vi "Example.vi"() -> ()   [LabVIEW 2021, in "Tree.lvlib"]
uses:
  Tree.lvlib
  Tree.lvclass
panel:
  in  "Show Hierarhy":T1={"Show hierarhy in first column(F)"=TRUE, "Left separator"="", "Right separator"="/"}
  in  "Column":i32=2
  in  "Clear":bool
  in  "InsertPath":bool
  in  "InsertClass":bool
  in  "InsertPane":bool
  out "Random to variant":dbl
  in  "Strings":string[](array[string])
  in  "Edit":bool
  out "Selected Element":T2
  in  "Variant":variant
  in  "InsertClaster":bool
  in  "Filter":string
  in  "StepForward":bool
  in  "StepBack":bool
  in  "Child?":bool
  in  "Delete":bool
  in  "New Tag":string
  in  "Strings":string[](array[string])
  in  "Add":bool
  in  "stop":bool
  in  "Tree":string[](tree)
  # "Tree v0.2"
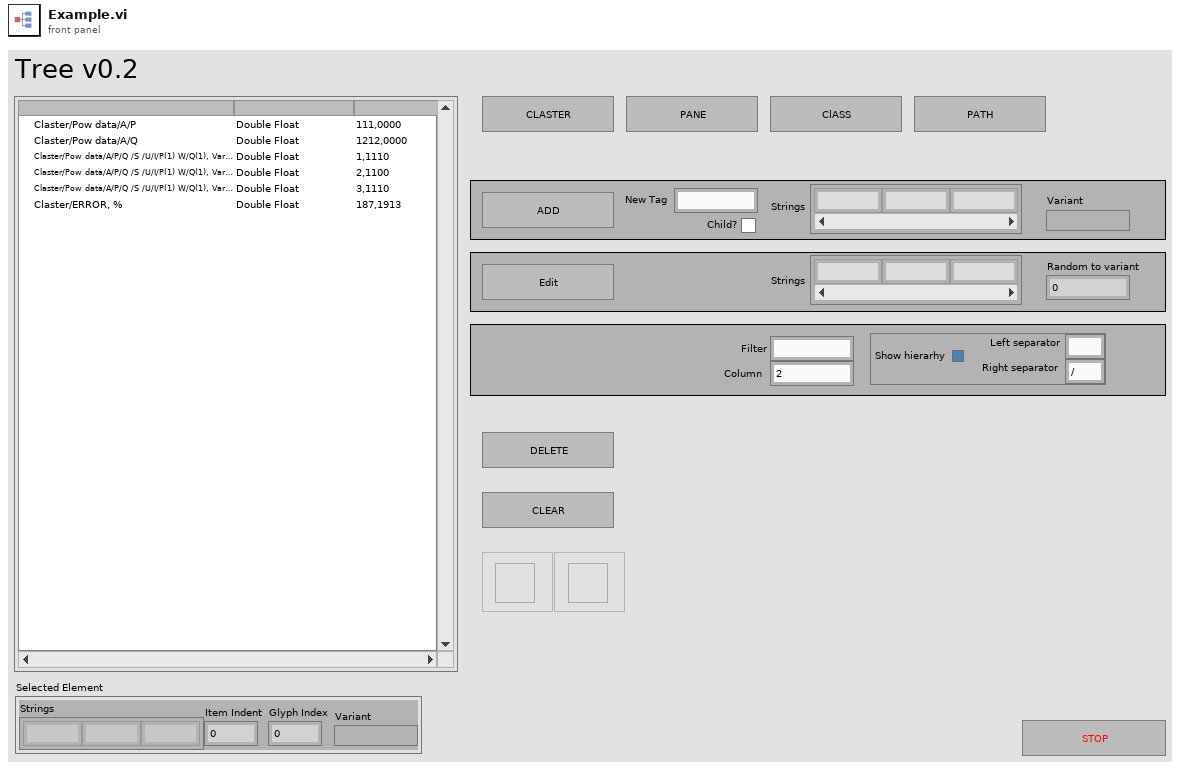
[diagram p1: front panel]
types:
  T1 = cluster{"Show hierarhy in first column(F)":bool, "Left separator":string, "Right separator":string}
  T2 = cluster{"Strings":string[], "Item Indent":i32, "Glyph Index":i32, "Variant":variant}
  T3 = enum16{"Clear & Insert", "Update Existing", "Add to End"}
  T4 = enum8{"Enabled", "Disabled", "Disabled and Grayed Out"}
  T5 = cluster{"Tag":string, "Strings":string[], "Open?":bool, "Item Indent":i32, "Glyph Index":i32, "Variant":variant}[]
  T6 = cluster{string, "New Tag":string, "Strings":string[], "Child?":bool, "Variant":variant}
  T7 = cluster{"Strings":string[], "Indent":i32, "Glyph Index":i32, "Variant":variant}
  T8 = cluster{"Pow data":cluster{"A":cluster{"P":dbl, "Q ":dbl, "S ":dbl, "U":dbl, "I":dbl, "P(1) W":dbl, "Q(1), Var":dbl, "S(1), VA":dbl, "cos(fi)":dbl, "sin(fi)":dbl, "Pow coef":string}, "B":cluster{"P":dbl, "Q ":dbl, "S ":dbl, "U":dbl, "I":dbl, "P(1) W":dbl, "Q(1), Var":dbl, "S(1), VA":dbl, "cos(fi)":dbl, "sin(fi)":dbl, "Pow coef":string}, "C":cluster{"P":dbl, "Q ":dbl, "S ":dbl, "U":dbl, "I":dbl, "P(1) W":dbl, "Q(1), Var":dbl, "S(1), VA":dbl, "cos(fi)":dbl, "sin(fi)":dbl, "Pow coef":string}, "N":cluster{"P":dbl, "Q ":dbl, "S ":dbl, "U":dbl, "I":dbl, "P(1) W":dbl, "Q(1), Var":dbl, "S(1), VA":dbl, "cos(fi)":dbl, "sin(fi)":dbl, "Pow coef":string}}, "Main data":cluster{"U":cluster{"RMS":cluster{"A":dbl, "B":dbl, "C":dbl, "N":dbl}, "DC":cluster{"A":dbl, "B":dbl, "C":dbl, "N":dbl}, "F(1)":cluster{"A":dbl, "B":dbl, "C":dbl, "N":dbl}, "RMS(1)":cluster{"A":dbl, "B":dbl, "C":dbl, "N":dbl}, "Phi":cluster{"A":dbl, "B":dbl, "C":dbl, "N":dbl}, "THD":cluster{"A":dbl, "B":dbl, "C":dbl, "N":dbl}}, "I":cluster{"RMS":cluster{"A":dbl, "B":dbl, "C":dbl, "N":dbl}, "DC":cluster{"A":dbl, "B":dbl, "C":dbl, "N":dbl}, "F(1)":cluster{"A":dbl, "B":dbl, "C":dbl, "N":dbl}, "RMS(1)":cluster{"A":dbl, "B":dbl, "C":dbl, "N":dbl}, "Phi":cluster{"A":dbl, "B":dbl, "C":dbl, "N":dbl}, "THD":cluster{"A":dbl, "B":dbl, "C":dbl, "N":dbl}}}, "Line voltage":cluster{"AB":dbl, "BC":dbl, "CA":dbl}, "Cref":dbl, "Nref_calc":dbl, "Ref Range":cluster{"I range":u8, "U range":u8}, "F out":cluster{"integer part":u32, "fractional part":u8}, "Ndut_culc_type":enum16{"Auto", "Ndut", "Tdut"}, "Ndut_calc":u32, "Tdut_calc":dbl, "ERROR, %":dbl, "Koef":u16, "Params 0xC5":cluster{"DUT_N":u32, "REF_N":u32, "REF_N 2":u32, "Iterations":u32}}
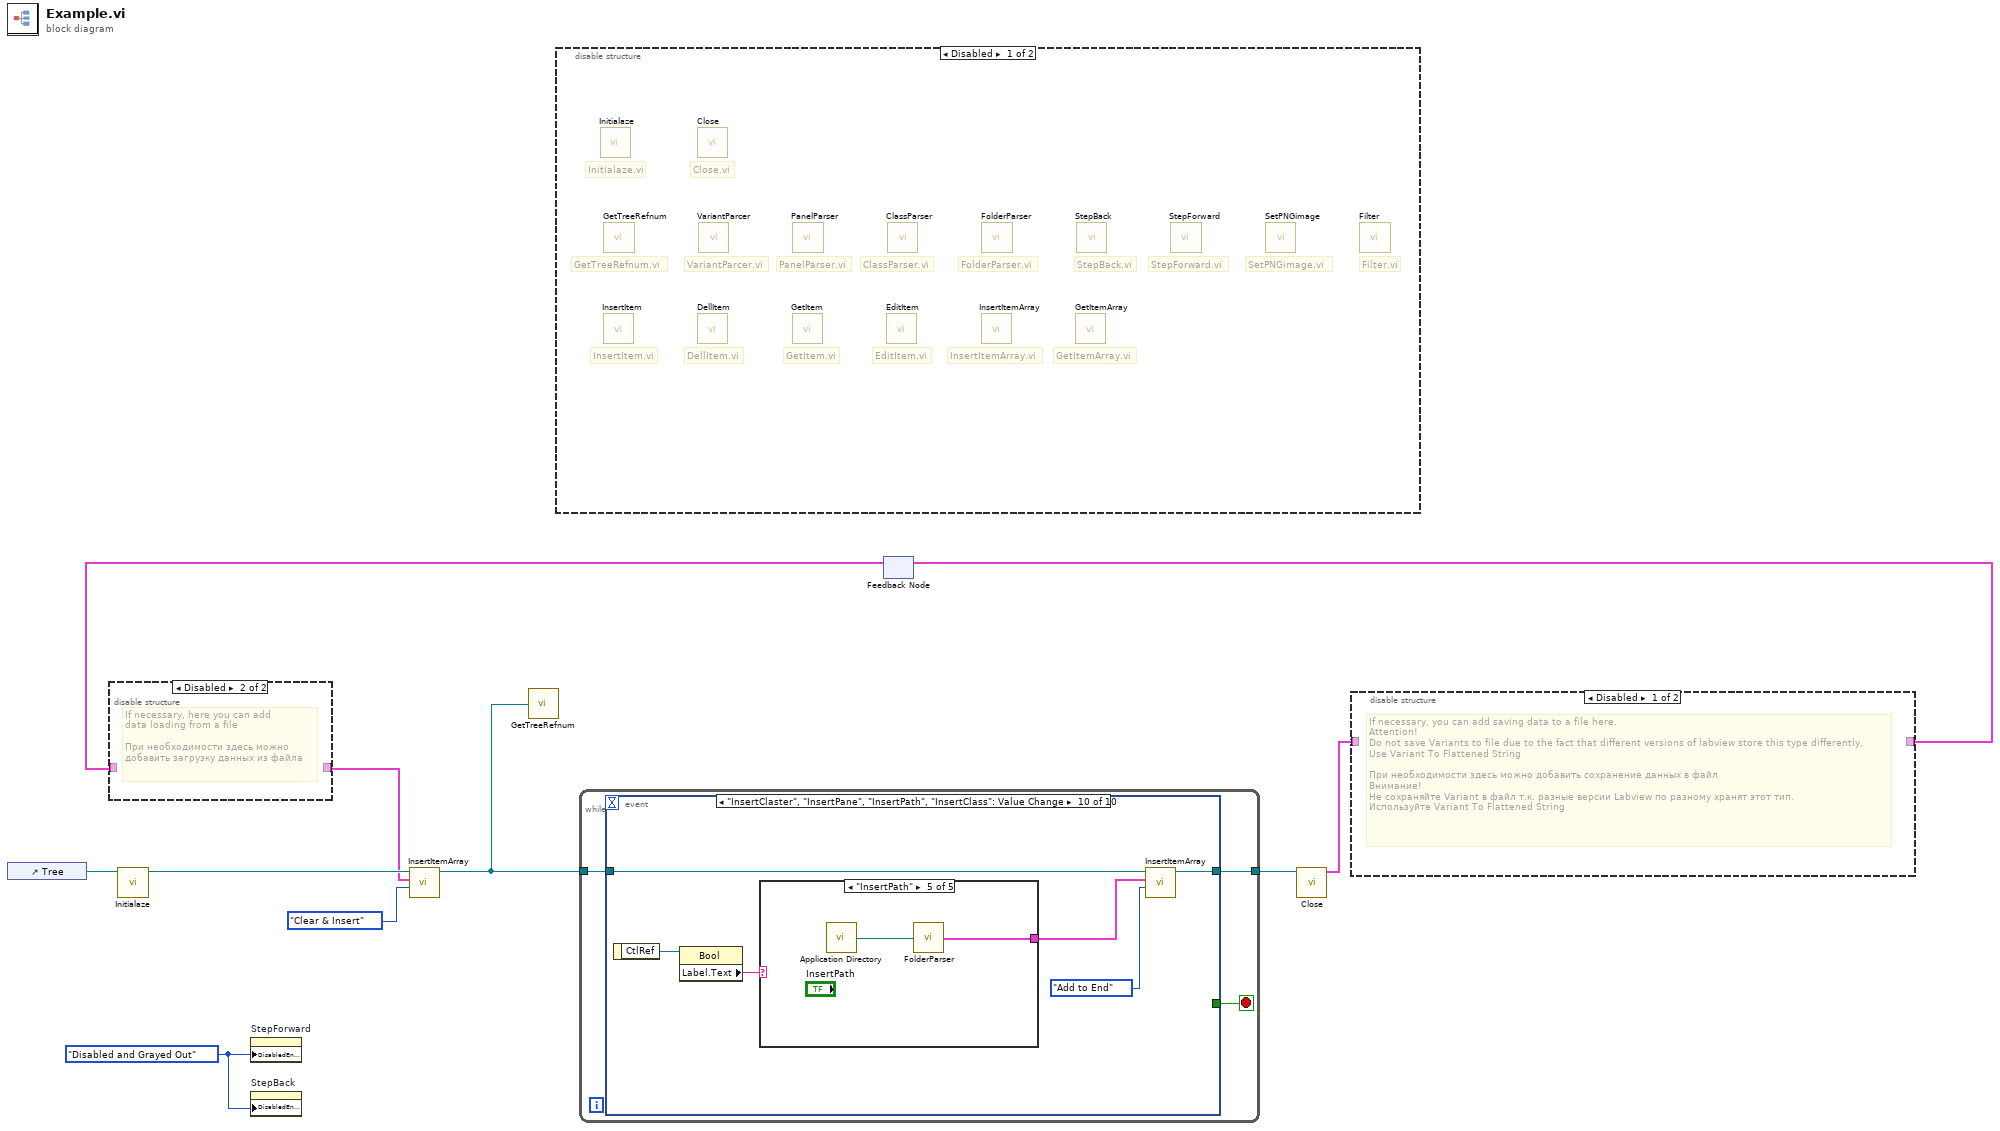
[diagram p0: block diagram]
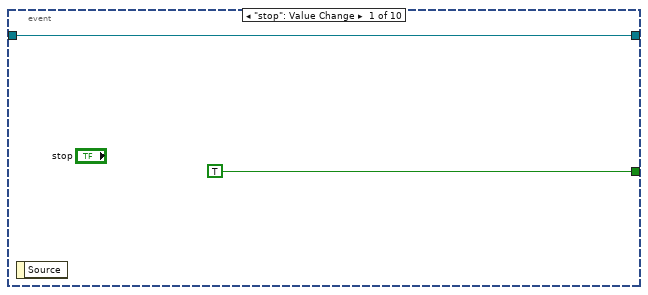
[diagram p5: hidden frame]
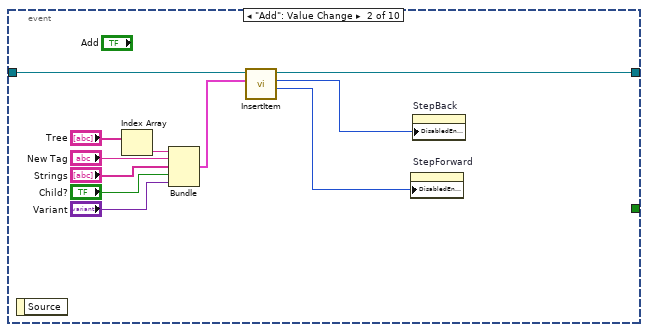
[diagram p6: hidden frame]
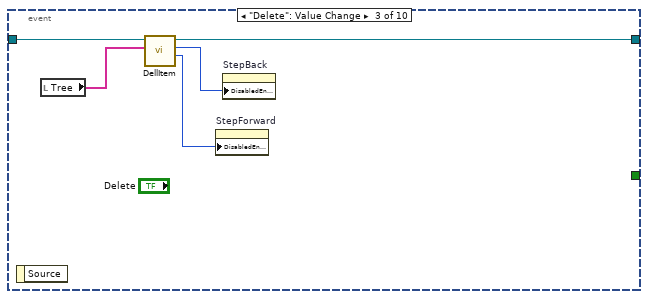
[diagram p7: hidden frame]
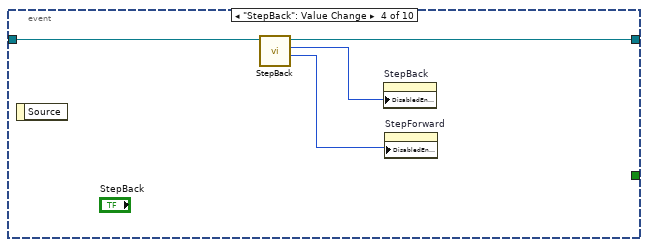
[diagram p8: hidden frame]
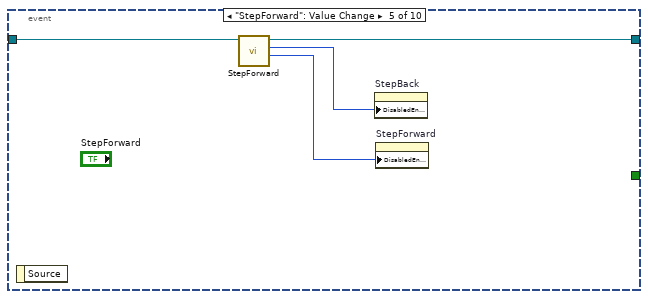
[diagram p9: hidden frame]
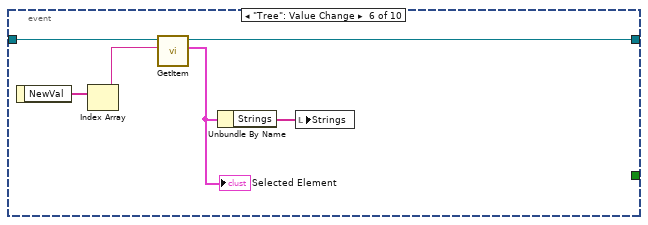
[diagram p10: hidden frame]
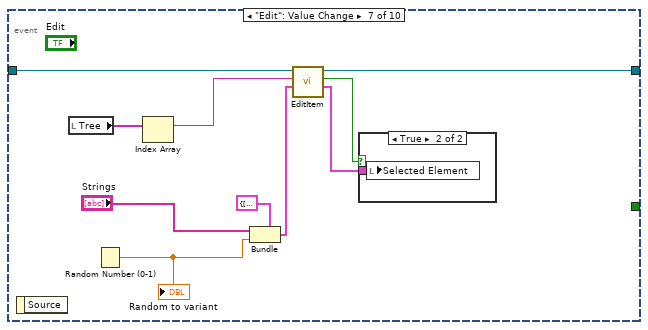
[diagram p11: hidden frame]
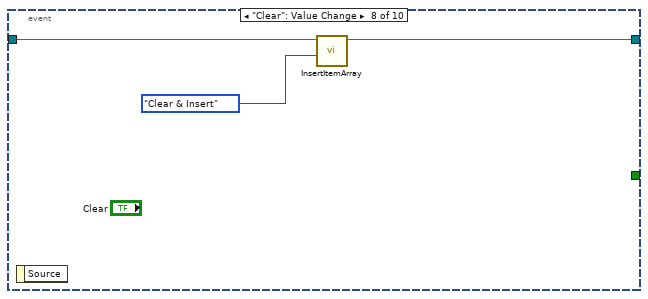
[diagram p13: hidden frame]
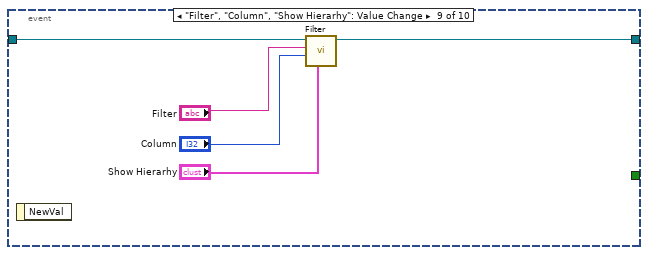
[diagram p14: hidden frame]
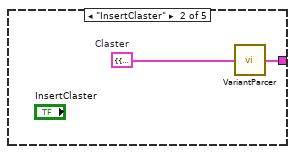
[diagram p16: hidden frame]
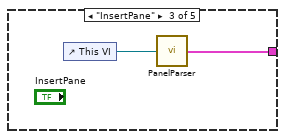
[diagram p17: hidden frame]
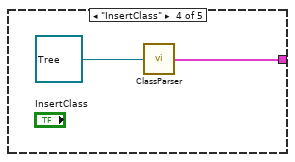
[diagram p18: hidden frame]
diagram:
  w3 = T4."Disabled and Grayed Out" ("Disabled")
  n1 = control-ref of="Tree"() -> (w10:refnum<vi>)
  n2 = call "Initialaze.vi"("Tree Refnum"=w10) -> ("TreeControl"=w7:refnum<class "Tree.lvclass">)  [unwired: 9 in, 1 out]
  n3 = property on="StepForward" class="Bool"("DisabledEnum"=w3) -> ()  [unwired: 2 in, 2 out]
  n4 = property on="StepBack" class="Bool"("DisabledEnum"=w3) -> ()  [unwired: 2 in, 2 out]
  n5 = disable-structure shown="Disabled" {
    frame Disabled {
      # "FolderParser.vi"
      # "ClassParser.vi"
      # "PanelParser.vi"
      # "Filter.vi"
      # "SetPNGimage.vi"
      # "EditItem.vi"
      # "InsertItem.vi"
      # "InsertItemArray.vi"
      # "GetItemArray.vi"
      # "StepForward.vi"
      # "StepBack.vi"
      # "GetItem.vi"
      # "DellItem.vi"
      # "Initialaze.vi"
      # "GetTreeRefnum.vi"
      # "VariantParcer.vi"
      # "Close.vi"
      n6 = call "Initialaze.vi"() -> ()  [unwired: 10 in, 2 out]
      n7 = call "InsertItem.vi"() -> ()  [unwired: 7 in, 5 out]
      n8 = call "GetTreeRefnum.vi"() -> ()  [unwired: 1 in, 1 out]
      n9 = call "Close.vi"() -> ()  [unwired: 9 in, 3 out]
      n10 = call "DellItem.vi"() -> ()  [unwired: 8 in, 4 out]
      n11 = call "VariantParcer.vi"() -> ()  [unwired: 1 in, 1 out]
      n12 = call "GetItem.vi"() -> ()  [unwired: 9 in, 3 out]
      n13 = call "PanelParser.vi"() -> ()  [unwired: 1 in, 1 out]
      n14 = call "EditItem.vi"() -> ()  [unwired: 8 in, 4 out]
      n15 = call "ClassParser.vi"() -> ()  [unwired: 1 in, 1 out]
      n16 = call "InsertItemArray.vi"() -> ()  [unwired: 10 in, 2 out]
      n17 = call "FolderParser.vi"() -> ()  [unwired: 1 in, 1 out]
      n18 = call "GetItemArray.vi"() -> ()  [unwired: 8 in, 4 out]
      n19 = call "StepBack.vi"() -> ()  [unwired: 8 in, 4 out]
      n20 = call "StepForward.vi"() -> ()  [unwired: 8 in, 4 out]
      n21 = call "SetPNGimage.vi"() -> ()  [unwired: 10 in, 2 out]
      n22 = call "Filter.vi"() -> ()  [unwired: 10 in, 2 out]
    }
    frame Enabled {
    }
  }
  n23 = feedback #1() -> (w6:T5)  [unwired: 1 in]
  n24 = disable-structure shown="Disabled" {
    disable-tunnel: [w11 _] -> w5
    disable-tunnel: w6 -> [w11 _]
    frame Enabled {
    }
    frame Disabled {
      # "If necessary, here you can add\ndata loading from a file\n\nПри необходимости здесь можно\nдобавить загрузку данных из файла"
    }
  }
  n25 = call "InsertItemArray.vi"("Mode"=T3."Clear & Insert", "TreeItems[]"=w5, "Tree in"=w7) -> ("Tree out"=w2:refnum<class "Tree.lvclass">)  [unwired: 7 in, 1 out]
  n26 = call "GetTreeRefnum.vi"("Tree in"=w2) -> ()  [unwired: 1 out]
  n27 = while {
    tunnel: w2 -> [w12]
    tunnel: [w13] -> w9
    stop <- w14 stop-if-true
    n28 = event shown="[9] \"InsertClaster\", \"InsertPane\", \"InsertPath\", \"InsertClass\": Value Change" {
      selector: _ -> [_ _ _ _ _ _ _ _ _ _]
      dyn-events: _ -> [_ _ _ _ _ _ _ _ _ _]
      timeout: _ -> [_ _ _ _ _ _ _ _ _ _]
      tunnel: [TRUE _ _ _ _ _ _ _ _ _] -> w14
      tunnel: [w15 w17 w28 w33 w37 w41 w50 w59 w64 w68] -> w13
      tunnel: w12 -> [w15 w27 w32 w36 w40 w46 w51 w60 w65 w71]
      event "stop": Value Change {
        n29 = event-data() -> ()  [unwired: 1 in, 1 out]
      }
      event "Add": Value Change {
        n30 = event-data() -> ()  [unwired: 1 in, 1 out]
        n31 = Index Array(array="Tree") -> (element=w24:string)  [unwired: 1 in]
        n32 = Bundle(w24, "New Tag"="New Tag", "Strings"="Strings", "Child?"="Child?", "Variant"="Variant") -> (w19:T6)  [unwired: 1 in]
        n33 = call "InsertItem.vi"("NewElement"=w19, "Tree in"=w27) -> ("StepForward"=w25:T4, "StepBack"=w26:T4, "Tree out"=w17:refnum<class "Tree.lvclass">)  [unwired: 5 in, 2 out]
        n34 = property on="StepForward" class="Bool"("DisabledEnum"=w25) -> ()  [unwired: 2 in, 2 out]
        n35 = property on="StepBack" class="Bool"("DisabledEnum"=w26) -> ()  [unwired: 2 in, 2 out]
      }
      event "Delete": Value Change {
        n36 = event-data() -> ()  [unwired: 1 in, 1 out]
        n37 = local read "Tree"() -> (w29:string[])
        n38 = call "DellItem.vi"("Tag"=w29, "Tree in"=w32) -> ("StepForward"=w30:T4, "StepBack"=w31:T4, "Tree out"=w28:refnum<class "Tree.lvclass">)  [unwired: 6 in, 1 out]
        n39 = property on="StepForward" class="Bool"("DisabledEnum"=w30) -> ()  [unwired: 2 in, 2 out]
        n40 = property on="StepBack" class="Bool"("DisabledEnum"=w31) -> ()  [unwired: 2 in, 2 out]
      }
      event "StepBack": Value Change {
        n41 = event-data() -> ()  [unwired: 1 in, 1 out]
        n42 = call "StepBack.vi"("Tree in"=w36) -> ("StepForward"=w34:T4, "StepBack"=w35:T4, "Tree out"=w33:refnum<class "Tree.lvclass">)  [unwired: 7 in, 1 out]
        n43 = property on="StepBack" class="Bool"("DisabledEnum"=w35) -> ()  [unwired: 2 in, 2 out]
        n44 = property on="StepForward" class="Bool"("DisabledEnum"=w34) -> ()  [unwired: 2 in, 2 out]
      }
      event "StepForward": Value Change {
        n45 = event-data() -> ()  [unwired: 1 in, 1 out]
        n46 = call "StepForward.vi"("Tree in"=w40) -> ("StepForward"=w38:T4, "StepBack"=w39:T4, "Tree out"=w37:refnum<class "Tree.lvclass">)  [unwired: 7 in, 1 out]
        n47 = property on="StepBack" class="Bool"("DisabledEnum"=w39) -> ()  [unwired: 2 in, 2 out]
        n48 = property on="StepForward" class="Bool"("DisabledEnum"=w38) -> ()  [unwired: 2 in, 2 out]
      }
      event "Tree": Value Change {
        n49 = event-data() -> ("NewVal"=w45:string[])  [unwired: 1 in]
        n50 = Index Array(array=w45) -> (element=w44:string)  [unwired: 1 in]
        n51 = call "GetItem.vi"("Tag"=w44, "Tree in"=w46) -> ("ItemData"=w43:T7, "Tree out"=w41:refnum<class "Tree.lvclass">)  [unwired: 7 in, 1 out]
        "Selected Element" <- w43
        n52 = Unbundle By Name(w43) -> ("Strings"=w42:string[])
        n53 = local write "Strings"(w42) -> ()
      }
      event "Edit": Value Change {
        n54 = event-data() -> ()  [unwired: 1 in, 1 out]
        n55 = local read "Tree"() -> (w56:string[])
        n56 = Random Number (0-1)() -> (number: 0 to 1=w52:dbl)
        "Random to variant" <- w52
        n57 = Index Array(array=w56) -> (element=w49:string)  [unwired: 1 in]
        n58 = Bundle(cluster=cluster{"Strings":string[], "Variant":variant} {"Strings"=[], "Variant"=variant} ("EditData"), "Strings"="Strings", "Variant"=w52) -> (w54:cluster{"Strings":string[], "Variant":variant})
        n59 = call "EditItem.vi"("EditData"=w54, "Tag"=w49, "Tree in"=w51) -> ("ItemData"=w48:T7, "Found?"=w47:bool, "Tree out"=w50:refnum<class "Tree.lvclass">)  [unwired: 5 in, 1 out]
        n60 = case shown="True" w47 {
          tunnel: w48 -> [_ w57]
          frame False {
          }
          frame True {
            n61 = local write "Selected Element"(w57) -> ()
          }
        }
      }
      event "Clear": Value Change {
        n62 = event-data() -> ()  [unwired: 1 in, 1 out]
        n63 = call "InsertItemArray.vi"("Mode"=T3."Clear & Insert", "Tree in"=w60) -> ("Tree out"=w59:refnum<class "Tree.lvclass">)  [unwired: 8 in, 1 out]
      }
      event "Filter", "Column", "Show Hierarhy": Value Change {
        n64 = event-data() -> ()  [unwired: 1 in, 1 out]
        n65 = call "Filter.vi"("Show Hierarhy"="Show Hierarhy", "Column"="Column", "Filter"="Filter", "Tree in"=w65) -> ("Tree out"=w64:refnum<class "Tree.lvclass">)  [unwired: 6 in, 1 out]
      }
      event "InsertClaster", "InsertPane", "InsertPath", "InsertClass": Value Change {
        n66 = event-data() -> ("CtlRef"=w67:refnum<vi>)  [unwired: 1 in]
        n67 = property class="Bool"(reference=w67) -> ("Label.Text"=w66:string)  [unwired: 1 in, 2 out]
        n68 = case shown="\"InsertPath\"" w66 {
          tunnel: [_ w73 w74 w76 w78] -> w70
          frame Default {
          }
          frame "InsertClaster" {
            w72 = T8 {"Pow data"={"A"={"P"=111.0, "Q "=1212.0, "S "=333.0, "U"=444.0, "I"=555.0, "P(1) W"=0.0, "Q(1), Var"=0.0, "S(1), VA"=0.0, "cos(fi)"=0.0, "sin(fi)"=0.0, "Pow coef"=""}, "B"={"P"=0.0, "Q "=0.0, "S "=0.0, "U"=0.0, "I"=0.0, "P(1) W"=0.0, "Q(1), Var"=0.0, "S(1), VA"=0.0, "cos(fi)"=0.0, "sin(fi)"=0.0, "Pow coef"=""}, "C"={"P"=0.0, "Q "=0.0, "S "=0.0, "U"=0.0, "I"=0.0, "P(1) W"=0.0, "Q(1), Var"=0.0, "S(1), VA"=0.0, "cos(fi)"=0.0, "sin(fi)"=0.0, "Pow coef"=""}, "N"={"P"=0.0, "Q "=0.0, "S "=0.0, "U"=0.0, "I"=0.0, "P(1) W"=0.0, "Q(1), Var"=0.0, "S(1), VA"=0.0, "cos(fi)"=0.0, "sin(fi)"=0.0, "Pow coef"=""}}, "Main data"={"U"={"RMS"={"A"=1.111, "B"=0.0, "C"=0.0, "N"=0.0}, "DC"={"A"=2.11, "B"=0.0, "C"=0.0, "N"=0.0}, "F(1)"={"A"=3.111, "B"=0.0, "C"=0.0, "N"=0.0}, "RMS(1)"={"A"=4.555, "B"=0.0, "C"=0.0, "N"=0.0}, "Phi"={"A"=5.0, "B"=0.0, "C"=0.0, "N"=0.0}, "THD"={"A"=0.0, "B"=0.0, "C"=0.0, "N"=0.0}}, "I"={"RMS"={"A"=0.0, "B"=0.0, "C"=0.0, "N"=0.0}, "DC"={"A"=0.0, "B"=0.0, "C"=0.0, "N"=0.0}, "F(1)"={"A"=0.0, "B"=0.0, "C"=0.0, "N"=0.0}, "RMS(1)"={"A"=0.0, "B"=0.0, "C"=0.0, "N"=0.0}, "Phi"={"A"=0.0, "B"=0.0, "C"=0.0, "N"=0.0}, "THD"={"A"=0.0, "B"=0.0, "C"=0.0, "N"=0.0}}}, "Line voltage"={"AB"=0.0, "BC"=0.0, "CA"=0.0}, "Cref"=0.0, "Nref_calc"=0.0, "Ref Range"={"I range"=6, "U range"=9}, "F out"={"integer part"=0, "fractional part"=0}, "Ndut_culc_type"=enum."Auto", "Ndut_calc"=0, "Tdut_calc"=0.0, "ERROR, %"=187.1912693854107, "Koef"=0, "Params 0xC5"={"DUT_N"=0, "REF_N"=0, "REF_N 2"=0, "Iterations"=0}}  # Claster
            n69 = call "VariantParcer.vi"("Variant"=w72) -> ("TreeItems[]"=w73:T5)
          }
          frame "InsertPane" {
            n70 = control-ref of="This VI"() -> (w75:refnum<vi>)
            n71 = call "PanelParser.vi"("VI reference"=w75) -> ("TreeItems[]"=w74:T5)
          }
          frame "InsertClass" {
            n72 = call "ClassParser.vi"("LabVIEW Object"=refnum<class "Tree.lvclass"> refnum ("TreeControl.lvlib:Tree.lvclass")) -> ("TreeItems[]"=w76:T5)
          }
          frame "InsertPath" {
            n73 = call <vilib>:"Application Directory.vi"() -> ("Application Directory"=w79:path)
            n74 = call "FolderParser.vi"("Folder"=w79) -> ("TreeItems[]"=w78:T5)
          }
        }
        n75 = call "InsertItemArray.vi"("Mode"=T3."Add to End", "TreeItems[]"=w70, "Tree in"=w71) -> ("Tree out"=w68:refnum<class "Tree.lvclass">)  [unwired: 7 in, 1 out]
      }
    }
  }
  n76 = call "Close.vi"("Tree in"=w9) -> ("TreeItems[]"=w4:T5)  [unwired: 8 in, 2 out]
  n77 = disable-structure shown="Disabled" {
    disable-tunnel: w4 -> [_ w80]
    disable-tunnel: [_ w80] -> w1
    frame Disabled {
      # "If necessary, you can add saving data to a file here.\nAttention!\nDo not save Variants to file due to the fact that different versions of labview store this type differently. \nUse Variant To Flattened String\n\nПри необходимости здесь можно добавить сохранение данных в файл \nВнимание!\nНе сохраняйте Variant в файл т.к. разные версии Labview по разному хранят этот тип. \nИспользуйте Variant To Flattened String"
    }
    frame Enabled {
    }
  }
  n78 = feedback-in #1(w1) -> ()
